vi "mlink_ao_write.vi"(6 "channels":u8[](array[numeric]), 7 "range":dbl[](array[numeric]), 8 "error in (no error)":errorcluster, 10 "data":dbl[](array[numeric]), 11 "connection ID":i32=-1) -> (0 "error out":errorcluster, 3 "connection ID out":i32)   [LabVIEW 2009, in "MicroDAQ.lvlib" / "mlink.lvlib"]
doc: "This function writes MicroDAQ analog outputs. The channels argument is an array containing channels numbers according to MicroDAQ hardware configuration. The ch_count argument determines number of used channels. The range argument specifies channel output range. An array n-by-2 where n is number of used channels shall be provided. In order to obtain \nsupported ranges check your analog output specification. The data argument points to array containing data to be set. The data array size must be same size as channels array and\nch_count parameter."
uses:
  <instrlib>/MicroDAQ/Mlink library wraper/mlink.lvlib
  <instrlib>/MicroDAQ/MLink32.dll
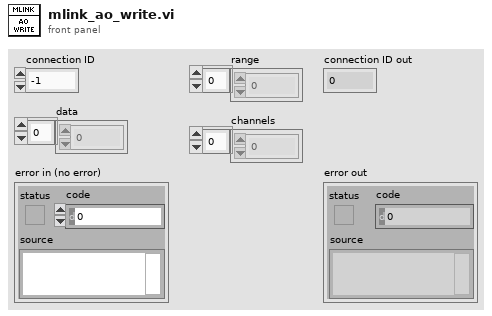
[diagram p1: front panel]
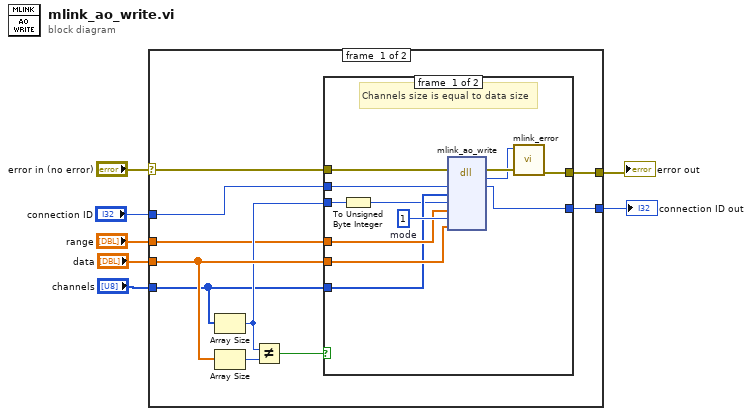
[diagram p0: block diagram]
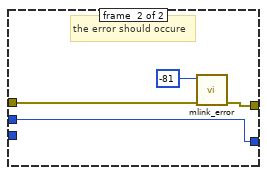
[diagram p2: hidden frame]
diagram:
  n1 = case shown="No Error" "error in (no error)" {
    selector: "error in (no error)" -> [w15 w35]
    tunnel: "connection ID" -> [w17 w34]
    tunnel: [w16 w34] -> w6
    tunnel: "data" -> [w14 _]
    tunnel: [w11 w35] -> w3
    tunnel: "range" -> [w9 _]
    tunnel: "channels" -> [w8 _]
    frame #0 {
      n2 = Array Size(array=w8) -> (size(s)=w12:i32)
      n3 = Array Size(array=w14) -> (size(s)=w13:i32)
      n4 = Not Equal?(x=w12, y=w13) -> (x != y?=w10:bool)
      n5 = case shown="False" w10 {
        tunnel: w17 -> [w29 w30]
        tunnel: [w28 w30] -> w16
        tunnel: w15 -> [w27 w32]
        tunnel: w14 -> [w25 _]
        tunnel: w12 -> [w24 _]
        tunnel: [w21 w33] -> w11
        tunnel: w9 -> [w20 _]
        tunnel: w8 -> [w19 _]
        frame #0 {
          w26 = u8 1  # mode
          # "Channels size is equal to data size"
          n6 = To Unsigned Byte Integer(number=w24) -> (unsigned 8bit integer=w18:u8)
          n7 = dll-call lib="C:/Program Files (x86)/National Instruments/LabVIEW 2009/instr.lib/MicroDAQ/MLink32.dll" fn="mlink_ao_write"(error in=w27, "link_fd"=w29, "ch"=w19, "ch_count"=w18, "range"=w20, "mode"=w26, "data"=w25) -> (error out=w23:errorcluster, "return type"=w22:i32, "link_fd"=w28:i32)  [unwired: 7 in, 1 out]
          n8 = call <instrlib>:"mlink_error.vi"("error in (no error)"=w23, "error code"=w22) -> ("error out"=w21:errorcluster)  [unwired: 9 in]
        }
        frame #1 {
          # "the error should occure"
          n9 = call <instrlib>:"mlink_error.vi"("error in (no error)"=w32, "error code"=-81 ("t")) -> ("error out"=w33:errorcluster)  [unwired: 9 in]
        }
      }
    }
    frame #1 {
    }
  }
  "connection ID out" <- w6
  "error out" <- w3
